vi "Diff_Drive_System_Get_AutoTuneCompleted.vi"() -> (1 "AutoTune Complete Right":bool, 3 "AutoTune Complete Left":bool)   [LabVIEW 2019]
uses:
  Diff_Drive_System_Globals.vi
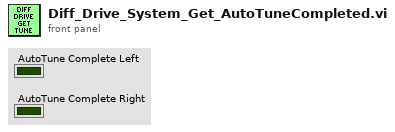
[diagram p1: front panel]
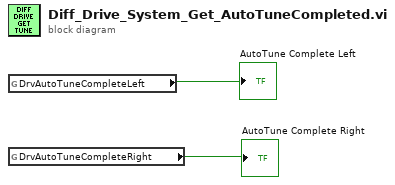
[diagram p0: block diagram]
diagram:
  n1 = global read "Diff_Drive_System_Globals.vi" "DrvAutoTuneCompleteLeft"() -> (→"AutoTune Complete Left":bool)
  n2 = global read "Diff_Drive_System_Globals.vi" "DrvAutoTuneCompleteRight"() -> (→"AutoTune Complete Right":bool)
